vi "prepractica 7.vi"() -> ()   [LabVIEW 2015]
panel:
  out "Promedio":dbl
  out "Mínimo":dbl
  out "Máximo":dbl
  out "Números aleatorios":dbl[](array[numeric])
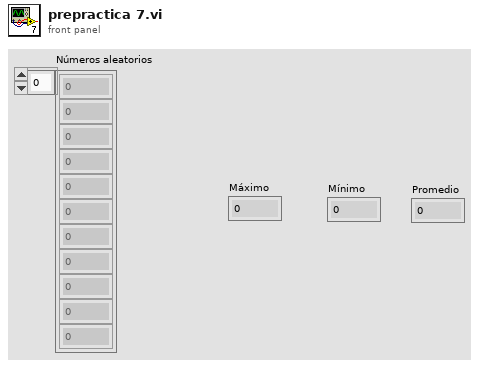
[diagram p1: front panel]
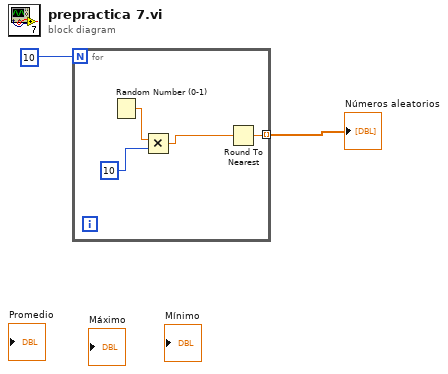
[diagram p0: block diagram]
diagram:
  n1 = for {
    N: 10 -> [_]
    tunnel: [w3] -> w1 mode=indexing
    n2 = Random Number (0-1) ("Random Number (-1,8-6,9)")() -> (number: 0 to 1=w6:dbl)
    n3 = Multiply(x=w6, y=10) -> (x*y=w4:dbl)
    n4 = Round To Nearest(number=w4) -> (nearest integer value=w3:dbl)
  }
  "Números aleatorios" <- w1
